vi "Read Attenuation.vi"(8 "error in":errorcluster, 11 "LTB-1 in":refnum<class "LTB-1.lvclass">) -> (0 "error out":errorcluster, 2 "Attenuation":dbl, 3 "LTB-1 out":refnum<class "LTB-1.lvclass">)   [LabVIEW 2018, in "LTB-1.lvlib" / "LTB-1.lvclass"]
doc: "This VI reads the current attenuation level. It will be overridden by the child class.\n\nThis can be used to confirm the attenuation value is within the specified range.\n\nAuthor: Ron Dexter\nCompany: Luminar\nModified: 5/20/2018"
uses:
  LTB-1.lvclass
  C:/AME Test Engineering/LabVIEW/PPLs/EXFO/Parent/EXFO.lvlibp/EXFO.lvclass
  LTB-1.lvclass/LTB-1.ctl
  PPLs/EXFO/Parent/EXFO.lvlibp/Methods/Read Resource.vi
  3150 Driver/3150.lvlib
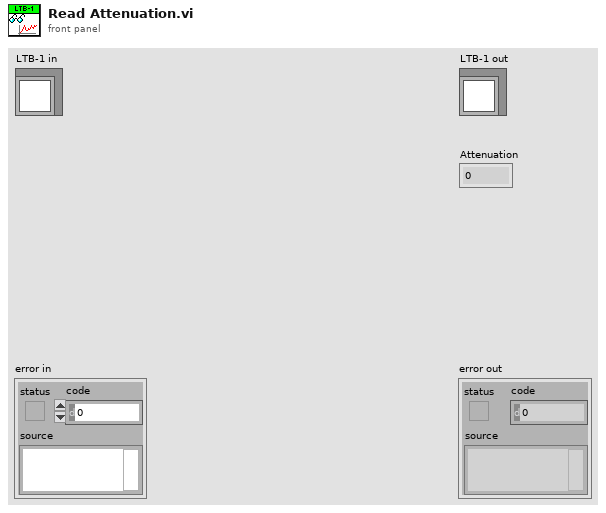
[diagram p1: front panel]
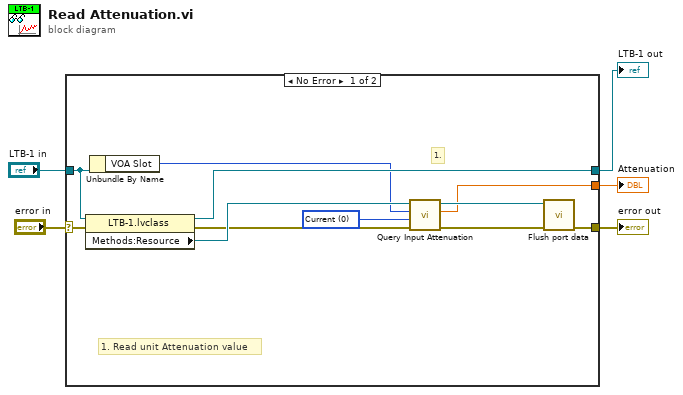
[diagram p0: block diagram]
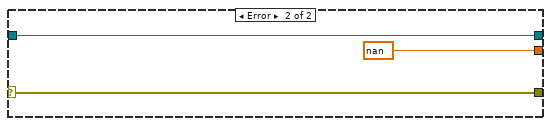
[diagram p2: hidden frame]
diagram:
  n1 = case shown="No Error" "error in" {
    selector: "error in" -> [w15 w17]
    tunnel: "LTB-1 in" -> [w13 w19]
    tunnel: [w16 w19] -> w4
    tunnel: [w14 w17] -> w3
    tunnel: [w8 nan ("Input Attenuation")] -> w2
    frame No Error {
      w9 = u16 0 items=["Current", "MINimum", "MAXimum", "DEFault"] ("Attenuation Type (0:Current)")
      # "1."
      # "1. Read unit Attenuation value"
      n2 = property class="LTB-1.lvclass"(reference=w13, error in=w15) -> (reference out=w16:refnum<class "LTB-1.lvclass">, error out=w6:errorcluster, "Methods:Resource"=w12:refnum<visa-resource-name>)
      n3 = Unbundle By Name(w13) -> ("VOA Slot"=w10:i16)
      n4 = call "Query Input Attenuation.vi"("error in (no error)"=w6, "Attenuation Type (0:Current)"=w9, "Platform Slot Number (10)"=w10, "VISA resource name"=w12) -> ("error out"=w7:errorcluster, "Input Attenuation"=w8:dbl, "VISA resource name out"=w11:refnum<visa-resource-name>)  [unwired: 5 in]
      n5 = call "Flush port data.vi"("error in (no error)"=w7, "VISA resource name"=w11) -> ("error out"=w14:errorcluster)  [unwired: 9 in]
    }
    frame Error {
    }
  }
  "error out" <- w3
  "LTB-1 out" <- w4
  "Attenuation" <- w2
